vi "PT3_Write.vi"(7 "Apend":bool=TRUE, 8 "error in":errorcluster, 9 "Data Count":i32, 10 "Data in":u32[](array[numeric]), 11 "refnum in":refnum<file>) -> (0 "error out":errorcluster, 3 "refnum out":refnum<file>)   [LabVIEW 2010]
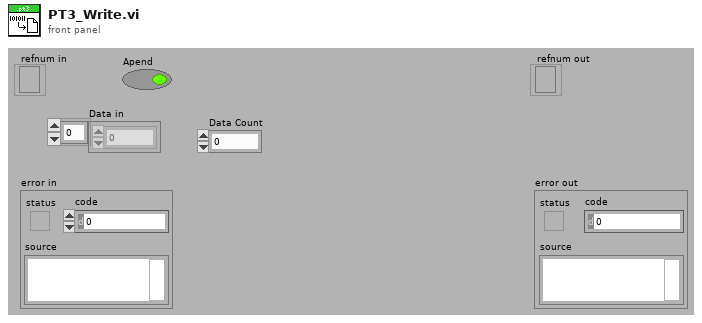
[diagram p1: front panel]
types:
  T1 = enum16{"big-endian, network order", "native, host order", "little-endian"}
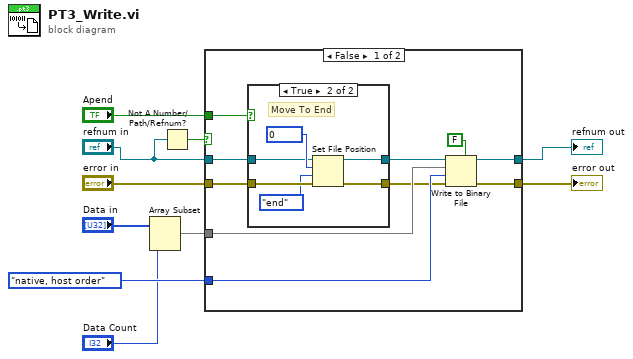
[diagram p0: block diagram]
diagram:
  n1 = Array Subset(array="Data in", length="Data Count") -> (w2:u32[])  [unwired: 1 in]
  n2 = Not A Number/Path/Refnum?(number/path/refnum="refnum in") -> (NaN/Path/Refnum?=w4:bool)
  n3 = case shown="False" w4 {
    tunnel: "error in" -> [w20 w30]
    tunnel: "refnum in" -> [w19 w29]
    tunnel: T1."native, host order" ("byte order (0:big-endian, network order)") -> [w18 _]
    tunnel: "Apend" -> [w17 _]
    tunnel: [w16 w29] -> w7
    tunnel: w2 -> [w15 _]
    tunnel: [w14 w30] -> w6
    frame False {
      n4 = case shown="True" w17 {
        tunnel: w20 -> [w22 w27]
        tunnel: w19 -> [w21 w26]
        tunnel: [w22 w24] -> w13
        tunnel: [w21 w23] -> w12
        frame False {
        }
        frame True {
          # "Move To End"
          n5 = Set File Position(offset (in bytes) (0)=i64 0, refnum=w26, from (0:start)=enum16{"start", "end", "current"}."end", error in=w27) -> (refnum out=w23:refnum<file>, error out=w24:errorcluster)
        }
      }
      n6 = Write to Binary File(file (use dialog)=w12, data=w15, error in=w13, 5:FALSE ("prepend array or string size? (T)"), 9:w18) -> (refnum out=w16:refnum<file>, error out=w14:errorcluster)  [unwired: 2 out]
    }
    frame True {
    }
  }
  "refnum out" <- w7
  "error out" <- w6
